vi "niDTS GNSS GPS Rx RF Test UTIL GPS to GNSS Parameters.vi"(1 "Parameters IN":T2 {"External Attenuation (dB)" format="%.1g"; "Power (dBm)" format="%.1g"}) -> (0 "Parameters OUT":T1={"GNSS Standard"=enum."GPS", "Frequency (Hz)"=0.0, "Auto Level"=FALSE, "Power (dBm)"=0.0, "External Attenuation (dB)"=0.0, "Measurement Interval (s)"=1000.0, "Pattern"=enum."PN9", "Enable Averaging"=FALSE, "Type Of Averaging"=enum."MEAN", "Number of Averages"=0, "Waveform Name"="", "Enable Traces"=FALSE} {"External Attenuation (dB)" format="%.1g"; "Power (dBm)" format="%.1g"})   [LabVIEW 2014, in "niDTS GNSS.lvlib"]
uses:
  niDTS GNSS.lvlib
  Includes/niDTS GNSS GPS Rx RF Test INC Parameters.ctl
  Includes/niDTS GNSS GPS Rx RF Test INC Channel.ctl
  RF Test/Includes/niDTS GNSS RF Test INC Parameters.ctl
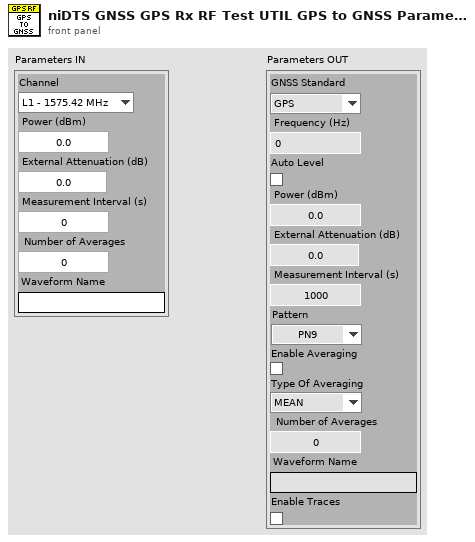
[diagram p1: front panel]
types:
  T1 = typedef "niDTS GNSS.lvlib/niDTS GNSS RF Test INC Parameters.ctl" = cluster{"GNSS Standard":enum16{"GPS", "GLONASS", "Galileo", "Beidou"}, "Frequency (Hz)":dbl, "Auto Level":bool, "Power (dBm)":dbl, "External Attenuation (dB)":dbl, "Measurement Interval (s)":dbl, "Pattern":enum16{"0", "1", "01", "00001111", "PN9"}, "Enable Averaging":bool, "Type Of Averaging":enum16{"MEAN", "MAX", "MIN", "MAXMIN"}, "Number of Averages":i32, "Waveform Name":string, "Enable Traces":bool}
  T2 = typedef "niDTS GNSS.lvlib/niDTS GNSS GPS Rx RF Test INC Parameters.ctl" = cluster{"Channel":T3, "Power (dBm)":dbl, "External Attenuation (dB)":dbl, "Measurement Interval (s)":dbl, "Number of Averages":i32, "Waveform Name":string}
  T3 = typedef "niDTS GNSS.lvlib/niDTS GNSS GPS Rx RF Test INC Channel.ctl" = enum16{"L1 - 1575.42 MHz", "L2 - 1227.60 MHz", "L5 - 1176.45 MHz"}
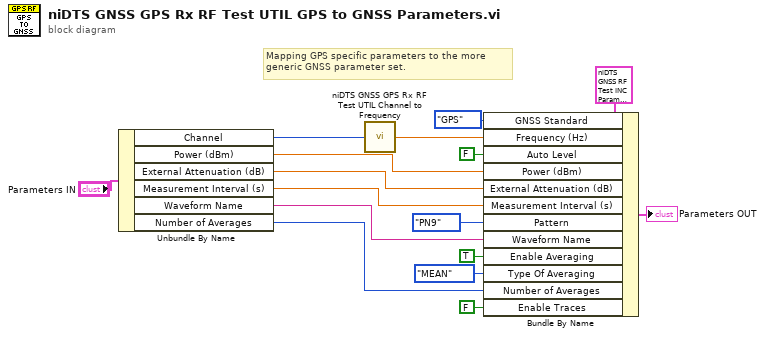
[diagram p0: block diagram]
diagram:
  # "Mapping GPS specific parameters to the more \ngeneric GNSS parameter set."
  n1 = Unbundle By Name("Parameters IN") -> ("Channel"=w9:T3, "Power (dBm)"=w10:dbl, "External Attenuation (dB)"=w12:dbl, "Measurement Interval (s)"=w6:dbl, "Waveform Name"=w7:string, "Number of Averages"=w5:i32)
  n2 = call "niDTS GNSS GPS Rx RF Test UTIL Channel to Frequency.vi"("Channel IN"=w9) -> ("Frequency (Hz) OUT"=w8:dbl)
  n3 = Bundle By Name(cluster=T1 {"GNSS Standard"=enum."GPS", "Frequency (Hz)"=0.0, "Auto Level"=FALSE, "Power (dBm)"=0.0, "External Attenuation (dB)"=0.0, "Measurement Interval (s)"=1000.0, "Pattern"=enum."PN9", "Enable Averaging"=FALSE, "Type Of Averaging"=enum."MEAN", "Number of Averages"=0, "Waveform Name"="", "Enable Traces"=FALSE} ("Parameters OUT"), "GNSS Standard"=enum16{"GPS", "GLONASS", "Galileo", "Beidou"}."GPS", "Frequency (Hz)"=w8, "Auto Level"=FALSE, "Power (dBm)"=w10, "External Attenuation (dB)"=w12, "Measurement Interval (s)"=w6, "Pattern"=enum16{"0", "1", "01", "00001111", "PN9"}."PN9", "Waveform Name"=w7, "Enable Averaging"=TRUE, "Type Of Averaging"=enum16{"MEAN", "MAX", "MIN", "MAXMIN"}."MEAN", "Number of Averages"=w5, "Enable Traces"=FALSE) -> (→"Parameters OUT":T1)
